vi "Timer Strategy.vi"() -> ()   [LabVIEW 2010]
panel:
  out "Waveform Chart":dbl(graph)
  out "Profit":dbl
  in  "Daily Balance":dbl
  in  "Daily Interest Gained":dbl
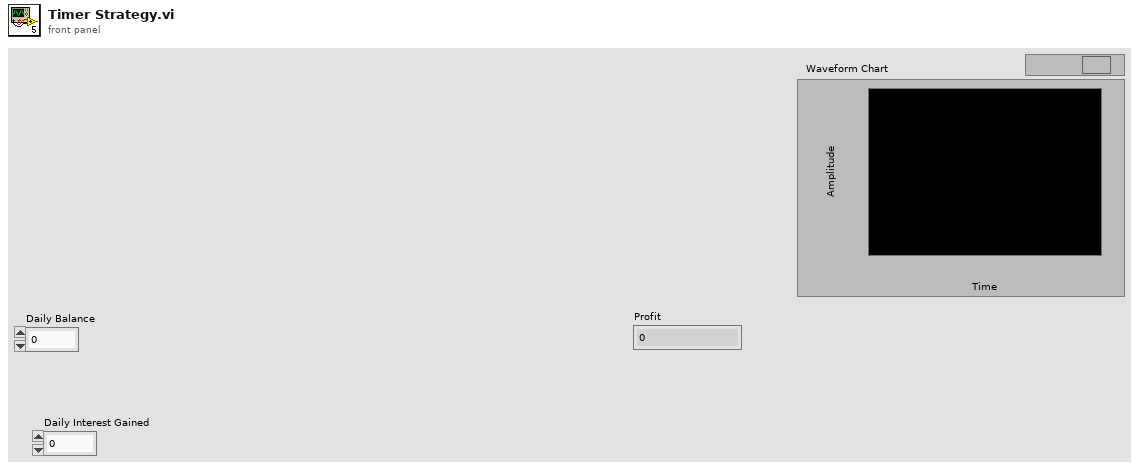
[diagram p1: front panel]
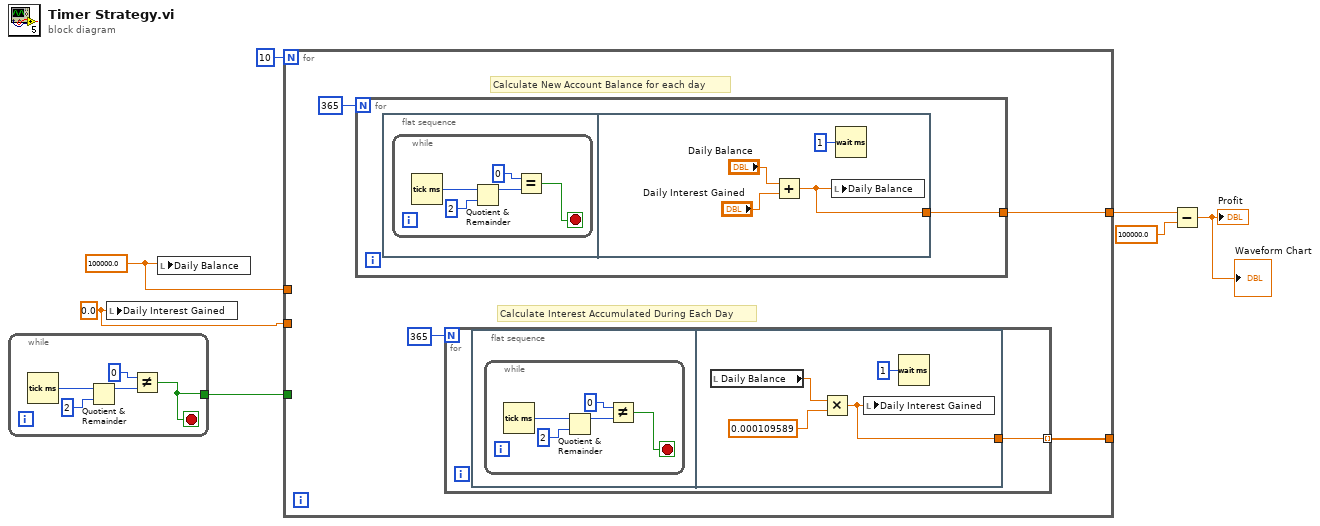
[diagram p0: block diagram]
diagram:
  w2 = 0.0 ("Daily Interest Gained")
  w3 = 100000.0 ("Daily Balance")
  n1 = while {
    tunnel: [w8] -> w4
    stop <- w8 stop-if-true
    n2 = Tick Count (ms)() -> (millisecond timer value=w12:u32)
    n3 = Quotient & Remainder(x=w12, y=u32 2) -> (x-y*floor(x/y)=w10:u32)  [unwired: 1 out]
    n4 = Not Equal?(x=u32 0, y=w10) -> (x != y?=w8:bool)
  }
  n5 = local write "Daily Interest Gained"(w2) -> ()
  n6 = local write "Daily Balance"(w3) -> ()
  n7 = for {
    N: 10 -> [_]
    tunnel: [w14] -> w6
    tunnel: w4 -> [_]
    tunnel: w3 -> [_]
    tunnel: w2 -> [_]
    tunnel: [w13] -> _
    # "Calculate Interest Accumulated During Each Day"
    # "Calculate New Account Balance for each day"
    n8 = for {
      N: 365 -> [_]
      tunnel: [w27] -> w14
      n9 = flat-sequence {
        tunnel: [w34] -> w27
        frame #0 {
          n10 = while {
            stop <- w28 stop-if-true
            n11 = Tick Count (ms)() -> (millisecond timer value=w32:u32)
            n12 = Quotient & Remainder(x=w32, y=u32 2) -> (x-y*floor(x/y)=w30:u32)  [unwired: 1 out]
            n13 = Equal?(x=u32 0, y=w30) -> (x = y?=w28:bool)
          }
        }
        frame #1 {
          n14 = Add(x="Daily Balance", y="Daily Interest Gained") -> (x+y=w34:dbl)
          n15 = local write "Daily Balance"(w34) -> ()
          n16 = Wait (ms)(milliseconds to wait=u32 1) -> ()  [unwired: 1 out]
        }
      }
    }
    n17 = for {
      N: 365 -> [_]
      tunnel: [w17] -> w13 mode=indexing
      n18 = flat-sequence {
        tunnel: [w24] -> w17
        frame #0 {
          n19 = while {
            stop <- w18 stop-if-true
            n20 = Tick Count (ms)() -> (millisecond timer value=w22:u32)
            n21 = Quotient & Remainder(x=w22, y=u32 2) -> (x-y*floor(x/y)=w20:u32)  [unwired: 1 out]
            n22 = Not Equal?(x=u32 0, y=w20) -> (x != y?=w18:bool)
          }
        }
        frame #1 {
          n23 = local read "Daily Balance"() -> (w26:dbl)
          n24 = Multiply(x=w26, y=0.000109589) -> (x*y=w24:dbl)
          n25 = local write "Daily Interest Gained"(w24) -> ()
          n26 = Wait (ms)(milliseconds to wait=u32 1) -> ()  [unwired: 1 out]
        }
      }
    }
  }
  n27 = Subtract(x=w6, y=100000.0) -> (x-y=→"Profit" →"Waveform Chart":dbl)
